vi "PickAndPlace_SiAndHB.vi"(0 "Operations":T1={"GoToTool"=TRUE, "PickTool"=TRUE, "GoToHB"=TRUE, "PickHB"=TRUE, "GoToSi"=TRUE, "PickSi"=TRUE, "GoToBP"=TRUE, "DropTool"=TRUE}, 1 "VacuumStates":path=path "C:/Users/TTUHEP/Documents/LabVIEW/GantryPrograms/Configs/PickPlaceVacuumStates.json", 5 "AssmbType":enum16{"BothSiHB", "Sensor", "HB"}(ring), 7 "Zone":enum16{"ZoneA", "ZoneB", "ZoneC", "ZoneD"}(ring), 9 "Position":enum16{"1", "2"}(ring), 11 "Error In":errorcluster) -> (4 "Log":string, 15 "Error Out":errorcluster)   [LabVIEW 2021]
panel:
  in  "Si Delay (milliseconds)":u32=30000
  in  "FastZHBPick":dbl=65.0
  out "HBXYZU":dbl[](array[numeric])
  out "Assembly_XYZU":dbl[](array[numeric])
  out "PUT_XYZU":dbl[](array[numeric])
  out "PUT rotation":dbl
  in  "FastZDrop":dbl=65.0
  in  "FastZToolPick":dbl=85.0
  in  "FastZSiPick":dbl=65.0
  in  "LineNo":u8
  in  "ZSpeed":dbl=10.0
  in  "XYSpeed":dbl=100.0
  out "SiXYZU":dbl[](array[numeric])
  out "ZoneBasedFileNameStarting":string
  in  "HB_PositionPartialFileName":string="HB_Position.txt"
  in  "SiPositionPartialFileName":string="Si_Position.txt"
  in  "PUT_PositionPartialFileName":string="PUT_Position.txt"
  in  "AssemblyPositionPartialFileName":string="BP_Position.txt"
  in  "BaseDirectory":string="C:\\Users\\TTUHEP\\Documents\\LabVIEW\\GantryPrograms\\Configs\\"
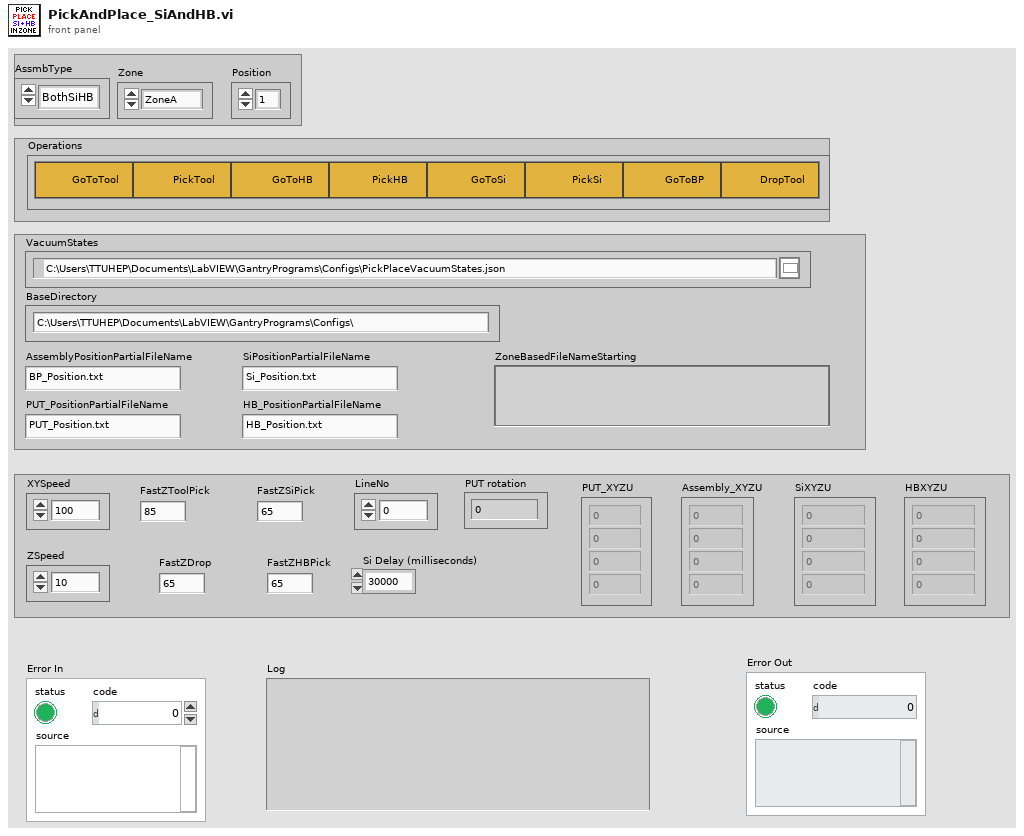
[diagram p1: front panel]
types:
  T1 = cluster{"GoToTool":bool, "PickTool":bool, "GoToHB":bool, "PickHB":bool, "GoToSi":bool, "PickSi":bool, "GoToBP":bool, "DropTool":bool}
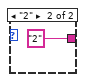
[diagram p2: hidden frame]
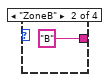
[diagram p3: hidden frame]
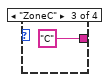
[diagram p4: hidden frame]
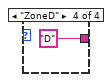
[diagram p5: hidden frame]
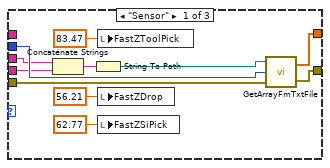
[diagram p6: hidden frame]
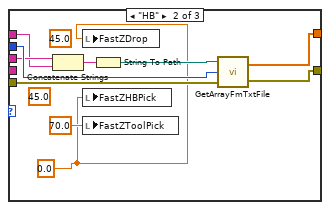
[diagram p7: hidden frame]
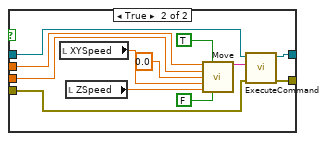
[diagram p8: hidden frame]
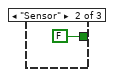
[diagram p10: hidden frame]
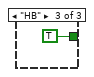
[diagram p11: hidden frame]
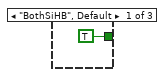
[diagram p14: hidden frame]
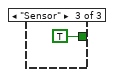
[diagram p15: hidden frame]
diagram:
  n1 = flat-sequence {
    tunnel: "Position" -> [w41]
    tunnel: "Zone" -> [w42]
    tunnel: [w42] -> w7
    tunnel: [w41] -> w6
    tunnel: [u8 0 ("LineNo")] -> w25
    tunnel: [w44] -> w17
    tunnel: ["Error In"] -> w16
    tunnel: w7 -> [w51]
    tunnel: w6 -> [w50]
    tunnel: [w64] -> w26
    tunnel: w25 -> [w63]
    tunnel: [w63] -> w23
    tunnel: w17 -> [w62]
    tunnel: w16 -> [w59]
    tunnel: [w118] -> w40
    tunnel: [w117] -> w39
    tunnel: [w116] -> w38
    tunnel: w26 -> [w114]
    tunnel: w23 -> [w115]
    tunnel: w40 -> [w145]
    tunnel: w39 -> [w144]
    tunnel: w38 -> [w143]
    tunnel: [w142] -> w37
    tunnel: [w141] -> w36
    tunnel: w37 -> [w151]
    tunnel: w36 -> [w150]
    tunnel: [w149] -> w35
    tunnel: [w148] -> w34
    tunnel: w35 -> [w189]
    tunnel: w34 -> [w188]
    tunnel: [w180] -> w5
    tunnel: [w179] -> w3
    tunnel: [w178] -> w2
    tunnel: [w215] -> w33
    tunnel: [w216] -> w32
    tunnel: w5 -> [w217]
    tunnel: [w217] -> w4
    tunnel: w3 -> [w216]
    tunnel: w2 -> [w215]
    tunnel: w33 -> [w225]
    tunnel: w32 -> [w224]
    tunnel: [w223] -> w11
    tunnel: [w222] -> w9
    tunnel: w4 -> [w220]
    tunnel: w11 -> [w262]
    tunnel: [w262] -> w10
    tunnel: w9 -> [w263]
    tunnel: [w263] -> w8
    tunnel: w10 -> [w272]
    tunnel: [w270] -> w15
    tunnel: w8 -> [w271]
    tunnel: [w269] -> w14
    tunnel: [w264] -> w1
    tunnel: w15 -> [w307]
    tunnel: w14 -> [w306]
    tunnel: [w303] -> w13
    tunnel: [w302] -> w12
    tunnel: w1 -> [w299]
    tunnel: w13 -> [w354]
    tunnel: [w352] -> w31
    tunnel: [w351] -> w30
    tunnel: [w350] -> w29
    tunnel: w12 -> [w355]
    tunnel: w31 -> [w382]
    tunnel: w30 -> [w381]
    tunnel: w29 -> [w379]
    tunnel: [w377] -> w28
    tunnel: [w376] -> w27
    tunnel: w28 -> [w388]
    tunnel: w27 -> [w387]
    tunnel: [w386] -> w21
    tunnel: [w385] -> w20
    tunnel: w21 -> [w426]
    tunnel: w20 -> [w425]
    tunnel: [w424] -> w18
    tunnel: [w431] -> w19
    tunnel: w18 -> [w429]
    frame #0 {
    }
    frame #1 {
      n2 = case shown="\"ZoneA\", Default" w51 {
        tunnel: ["A" "B" "C" "D"] -> w47
        frame "ZoneA", Default {
        }
        frame "ZoneB" {
        }
        frame "ZoneC" {
        }
        frame "ZoneD" {
        }
      }
      n3 = case shown="\"1\", Default" w50 {
        tunnel: ["1" "2"] -> w46
        frame "1", Default {
        }
        frame "2" {
        }
      }
      n4 = Concatenate Strings(w47, w46, "_" ("string")) -> (w49:string)
      n5 = Concatenate Strings("BaseDirectory", w49) -> (w44:string)
      "ZoneBasedFileNameStarting" <- w44
    }
    frame #2 {
      n6 = case shown="\"BothSiHB\", Default" "AssmbType" {
        tunnel: w63 -> [w77 w87 w92]
        tunnel: [w76 w86 w103] -> w66
        tunnel: w59 -> [w75 w85 w102]
        tunnel: [w74 w84 w90] -> w64
        tunnel: w62 -> [w70 w82 w94]
        tunnel: "SiPositionPartialFileName" -> [w67 _ w97]
        tunnel: "HB_PositionPartialFileName" -> [_ w79 w93]
        frame "Sensor" {
          n7 = Concatenate Strings(w70, w67) -> (w69:string)
          n8 = String To Path(string=w69) -> (path=w68:path)
          n9 = local write "FastZToolPick"(83.47 ("FastZToolPick")) -> ()
          n10 = local write "FastZDrop"(56.21 ("FastZDrop")) -> ()
          n11 = local write "FastZSiPick"(62.77 ("FastZSiPCBPick")) -> ()
          n12 = call "GetArrayFmTxtFile.vi"("error in"=w75, "LineNo."=w77, "TextFile"=w68) -> ("error out"=w74:errorcluster, "Array"=w76:dbl[])
        }
        frame "HB" {
          w78 = 0.0
          (unwired) 45.0 ("FastZDrop")
          (unwired) 45.0 ("FastZSiPCBPick")
          n13 = Concatenate Strings(w82, w79) -> (w81:string)
          n14 = local write "FastZDrop"(w78) -> ()
          n15 = local write "FastZHBPick"(w78) -> ()
          n16 = local write "FastZToolPick"(70.0 ("FastZToolPick")) -> ()
          n17 = String To Path(string=w81) -> (path=w80:path)
          n18 = call "GetArrayFmTxtFile.vi"("error in"=w85, "LineNo."=w87, "TextFile"=w80) -> ("error out"=w84:errorcluster, "Array"=w86:dbl[])
        }
        frame "BothSiHB", Default {
          w88 = 0.0
          (unwired) 45.0 ("FastZSiPCBPick")
          (unwired) 48.0 ("FastZDrop")
          n19 = Concatenate Strings(w94, w93) -> (w96:string)
          n20 = Concatenate Strings(w94, w97) -> (w99:string)
          n21 = local write "FastZSiPick"(60.0 ("FastZSiPCBPick")) -> ()
          n22 = local write "FastZToolPick"(80.0 ("FastZToolPick")) -> ()
          n23 = local write "FastZHBPick"(w88) -> ()
          n24 = local write "FastZDrop"(w88) -> ()
          n25 = String To Path(string=w96) -> (path=w95:path)
          n26 = String To Path(string=w99) -> (path=w98:path)
          n27 = call "GetArrayFmTxtFile.vi"("error in"=w102, "LineNo."=w92, "TextFile"=w98) -> ("error out"=w91:errorcluster, "Array"=w103:dbl[])
          n28 = call "GetArrayFmTxtFile.vi"("error in"=w91, "LineNo."=w92, "TextFile"=w95) -> ("error out"=w90:errorcluster, "Array"=→"HBXYZU":dbl[])
        }
      }
      "SiXYZU" <- w66
    }
    frame #3 {
      n29 = local read "ZoneBasedFileNameStarting"() -> (w110:string)
      n30 = Concatenate Strings(w110, "PUT_PositionPartialFileName") -> (w109:string)
      n31 = String To Path(string=w109) -> (path=w108:path)
      n32 = call "GetArrayFmTxtFile.vi"("error in"=w114, "LineNo."=w115, "TextFile"=w108) -> ("error out"=w107:errorcluster, "Array"=w112:dbl[])
      "PUT_XYZU" <- w112
      n33 = local read "Operations"() -> (w105:T1)
      n34 = call "Connect.vi"("error in (no error)"=w107) -> ("error out"=w106:errorcluster, "controller"=w113:refnum<k24>)  [unwired: 9 in]
      n35 = Index Array(array=w112, index=3) -> (element=w116:dbl)
      "PUT rotation" <- w116
      n36 = Index Array(array=w112, index=0) -> (element=w120:dbl)
      n37 = Index Array(array=w112, index=1) -> (element=w119:dbl)
      n38 = Unbundle By Name(w105) -> ("GoToTool"=w104:bool)
      n39 = call "ExecuteCommand.vi"("error in (no error)"=w106, "Command Code"="G90\nG1 Z0 F50", "controller in"=w113) -> ("error out"=w126:errorcluster, "controller out"=w125:refnum<k24>)  [unwired: 6 in, 1 out]
      n40 = case shown="False" w104 {
        tunnel: w125 -> [w128 w137]
        tunnel: w126 -> [w127 w136]
        tunnel: [w127 w135] -> w118
        tunnel: [w128 w134] -> w117
        tunnel: w120 -> [_ w133]
        tunnel: w119 -> [_ w132]
        frame False {
        }
        frame True {
          n41 = local read "XYSpeed"() -> (w130:dbl)
          n42 = local read "ZSpeed"() -> (w129:dbl)
          n43 = call "Move.vi"("X"=w133, "Absolute"=TRUE, "Y"=w132, "Z"=0.0, "SpeedXY (mm/s)"=w130, "SpeedZ (mm/s)"=w129, "Move Z first"=FALSE) -> ("Position Gcode"=w138:string)  [unwired: 8 in]
          n44 = call "ExecuteCommand.vi"("error in (no error)"=w136, "Command Code"=w138, "controller in"=w137) -> ("error out"=w135:errorcluster, "controller out"=w134:refnum<k24>)  [unwired: 6 in, 1 out]
        }
      }
    }
    frame #4 {
      n45 = call "RotateGH_U.vi"("error in (no error)"=w145, "controller in"=w144, "U"=w143) -> ("error out"=w142:errorcluster, "controller out"=w141:refnum<k24>)
    }
    frame #5 {
      n46 = local read "Operations"() -> (w146:T1)
      n47 = Unbundle By Name(w146) -> ("PickTool"=w147:bool)
      n48 = case shown="True" w147 {
        tunnel: w151 -> [w153 w162]
        tunnel: w150 -> [w152 w175]
        tunnel: [w153 w154] -> w149
        tunnel: [w152 w158] -> w148
        frame False {
        }
        frame True {
          w165 = u8 0
          n49 = call "JSONfileReader.vi"("error in"=w162, "Variant"=w165, "ItemName"="PickTool", "FileIn"="VacuumStates") -> ("error out"=w160:errorcluster, "Data"=w164:variant, "Found"=w169:bool)
          n50 = Not(x=w169) -> (.not. x?=w170:bool)
          n51 = Variant To Data(error in=w160, type=w165, Variant=w164) -> (data=w163:u8, error out=w159:errorcluster)
          n52 = local read "FastZToolPick"() -> (w157:dbl)
          n53 = local read "Position"() -> (w174:enum16{"1", "2"})
          n54 = call "AddError.vi"("NoErrorMessage"="Vac OK", "ErrorMessage"="Could not get vacuum state from json file.", "error in"=w159, "code"=-998, "Error?"=w170) -> ("Error out"=w161:errorcluster)  [unwired: 6 in]
          n55 = local read "Zone"() -> (w173:enum16{"ZoneA", "ZoneB", "ZoneC", "ZoneD"})
          n56 = call "ZoneVacCtrldPickDrop.vi"("Position"=w174, "Zone"=w173, "VacuumState"=w163, "error in (no error)"=w161, "controller in"=w175, "Zspeed"=50.0, "Z"=w157) -> ("error out"=w155:errorcluster, "controller out"=w158:refnum<k24>)  [unwired: 3 in]
          n57 = call <vilib>:"Simple Error Handler.vi"("error in (no error)"=w155) -> ("error?"=w156:bool, "error out"=w154:errorcluster)  [unwired: 4 in, 3 out]
          n58 = Stop(stop? (T)=w156) -> ()
        }
      }
    }
    frame #6 {
      n59 = local read "AssmbType"() -> (w183:enum16{"BothSiHB", "Sensor", "HB"})
      n60 = case shown="\"BothSiHB\", Default" w183 {
        tunnel: [TRUE FALSE TRUE] -> w180
        frame "BothSiHB", Default {
        }
        frame "Sensor" {
        }
        frame "HB" {
        }
      }
      n61 = local read "Operations"() -> (w184:T1)
      n62 = local read "HBXYZU"() -> (w187:dbl[])
      n63 = local read "PUT rotation"() -> (w186:dbl)
      n64 = Unbundle By Name(w184) -> ("GoToHB"=w182:bool)
      n65 = Index Array(array=w187, index=3) -> (element=w185:dbl)
      n66 = Index Array(array=w187, index=0) -> (element=w193:dbl)
      n67 = Index Array(array=w187, index=1) -> (element=w194:dbl)
      n68 = Add(x=w186, y=w185) -> (x+y=w177:dbl)
      n69 = And(x=w182, y=w180) -> (x .and. y?=w181:bool)
      n70 = case shown="True" w181 {
        tunnel: w188 -> [w199 w211]
        tunnel: w189 -> [w198 w210]
        tunnel: w193 -> [_ w209]
        tunnel: w194 -> [_ w208]
        tunnel: [w198 w204] -> w179
        tunnel: [w199 w203] -> w178
        tunnel: w177 -> [_ w202]
        frame False {
        }
        frame True {
          n71 = local read "XYSpeed"() -> (w205:dbl)
          n72 = local read "ZSpeed"() -> (w206:dbl)
          n73 = call "Move.vi"("X"=w209, "Absolute"=TRUE, "Y"=w208, "Z"=0.0, "SpeedXY (mm/s)"=w205, "SpeedZ (mm/s)"=w206, "Move Z first"=FALSE) -> ("Position Gcode"=w212:string)  [unwired: 8 in]
          n74 = call "ExecuteCommand.vi"("error in (no error)"=w210, "Command Code"=w212, "controller in"=w211) -> ("error out"=w200:errorcluster, "controller out"=w201:refnum<k24>)  [unwired: 6 in, 1 out]
          n75 = call "RotateGH_U.vi"("error in (no error)"=w200, "controller in"=w201, "U"=w202) -> ("error out"=w204:errorcluster, "controller out"=w203:refnum<k24>)
        }
      }
    }
    frame #7 {
    }
    frame #8 {
      n76 = local read "Operations"() -> (w221:T1)
      n77 = Unbundle By Name(w221) -> ("PickHB"=w218:bool)
      n78 = And(x=w220, y=w218) -> (x .and. y?=w219:bool)
      n79 = case shown="True" w219 {
        tunnel: w224 -> [w227 w248]
        tunnel: w225 -> [w226 w242]
        tunnel: [w227 w245] -> w222
        tunnel: [w226 w244] -> w223
        frame False {
        }
        frame True {
          w236 = u8 0
          w251 = u8 0
          w229 = "Could not get vacuum state from json file." ("ErrorMessage")
          n80 = local read "VacuumStates"() -> (w232:path)
          n81 = call "JSONfileReader.vi"("error in"=w248, "Variant"=w251, "ItemName"="PickHB", "FileIn"=w232) -> ("error out"=w247:errorcluster, "Data"=w250:variant, "Found"=w254:bool)
          n82 = Not(x=w254) -> (.not. x?=w255:bool)
          n83 = Variant To Data(error in=w247, type=w251, Variant=w250) -> (data=w249:u8, error out=w246:errorcluster)
          n84 = call "AddError.vi"("NoErrorMessage"="Vac OK", "ErrorMessage"=w229, "error in"=w246, "code"=-998, "Error?"=w255) -> ("Error out"=w231:errorcluster)  [unwired: 6 in]
          n85 = call "JSONfileReader.vi"("error in"=w231, "Variant"=w236, "ItemName"="ReleaseHB", "FileIn"=w232) -> ("error out"=w234:errorcluster, "Data"=w235:variant, "Found"=w239:bool)
          n86 = Not(x=w239) -> (.not. x?=w240:bool)
          n87 = Variant To Data(error in=w234, type=w236, Variant=w235) -> (data=w228:u8, error out=w233:errorcluster)
          n88 = local read "FastZHBPick"() -> (w243:dbl)
          n89 = local read "Position"() -> (w258:enum16{"1", "2"})
          n90 = call "AddError.vi"("NoErrorMessage"="Vac OK", "ErrorMessage"=w229, "error in"=w233, "code"=-998, "Error?"=w240) -> ("Error out"=w230:errorcluster)  [unwired: 6 in]
          n91 = local read "Zone"() -> (w257:enum16{"ZoneA", "ZoneB", "ZoneC", "ZoneD"})
          n92 = call "ZoneVacCtrldPickDrop_2StepVac.vi"("Position"=w258, "VacuumState2"=w228, "Zone"=w257, "VacuumState1"=w249, "error in (no error)"=w230, "controller in"=w242, "Zspeed"=50.0, "Z"=w243) -> ("error out"=w245:errorcluster, "controller out"=w244:refnum<k24>)  [unwired: 2 in]
        }
      }
    }
    frame #9 {
      n93 = One Button Dialog(message="Removed tape on HB?", button name ("OK")="Yes" ("T button name (\"OK\")")) -> ()  [unwired: 1 out]
    }
    frame #10 {
      n94 = local read "AssmbType"() -> (w267:enum16{"BothSiHB", "Sensor", "HB"})
      n95 = local read "Operations"() -> (w268:T1)
      n96 = case shown="\"HB\"" w267 {
        tunnel: [TRUE FALSE TRUE] -> w265
        frame "BothSiHB", Default {
        }
        frame "HB" {
        }
        frame "Sensor" {
        }
      }
      n97 = Unbundle By Name(w268) -> ("GoToSi"=w266:bool)
      n98 = And(x=w266, y=w265) -> (x .and. y?=w264:bool)
      n99 = case shown="True" w264 {
        tunnel: w272 -> [w277 w289]
        tunnel: w271 -> [w276 w288]
        tunnel: [w277 w284] -> w270
        tunnel: [w276 w283] -> w269
        frame False {
        }
        frame True {
          n100 = local read "SiXYZU"() -> (w279:dbl[])
          n101 = local read "PUT rotation"() -> (w278:dbl)
          n102 = local read "XYSpeed"() -> (w281:dbl)
          n103 = local read "ZSpeed"() -> (w280:dbl)
          n104 = Index Array(array=w279, index=3) -> (element=w287:dbl)
          n105 = Index Array(array=w279, index=0) -> (element=w292:dbl)
          n106 = Index Array(array=w279, index=1) -> (element=w291:dbl)
          n107 = Add(x=w278, y=w287) -> (x+y=w286:dbl)
          n108 = call "Move.vi"("X"=w292, "Absolute"=TRUE, "Y"=w291, "Z"=0.0, "SpeedXY (mm/s)"=w281, "SpeedZ (mm/s)"=w280, "Move Z first"=FALSE) -> ("Position Gcode"=w296:string)  [unwired: 8 in]
          n109 = call "ExecuteCommand.vi"("error in (no error)"=w288, "Command Code"=w296, "controller in"=w289) -> ("error out"=w282:errorcluster, "controller out"=w285:refnum<k24>)  [unwired: 6 in, 1 out]
          n110 = call "RotateGH_U.vi"("error in (no error)"=w282, "controller in"=w285, "U"=w286) -> ("error out"=w283:errorcluster, "controller out"=w284:refnum<k24>)
        }
      }
    }
    frame #11 {
      n111 = local read "Operations"() -> (w304:T1)
      n112 = local read "VacuumStates"() -> (w305:path)
      n113 = Unbundle By Name(w304) -> ("PickSi"=w300:bool)
      n114 = And(x=w300, y=w299) -> (x .and. y?=w301:bool)
      n115 = case shown="True" w301 {
        tunnel: w306 -> [w309 w333]
        tunnel: w307 -> [w308 w328]
        tunnel: [w309 w330] -> w303
        tunnel: [w308 w329] -> w302
        tunnel: w305 -> [_ w314]
        frame False {
        }
        frame True {
          w322 = u8 0
          w336 = u8 0
          w316 = "Could not get vacuum state from json file." ("ErrorMessage")
          n116 = call "JSONfileReader.vi"("error in"=w333, "Variant"=w336, "ItemName"="PickSi", "FileIn"=w314) -> ("error out"=w332:errorcluster, "Data"=w335:variant, "Found"=w339:bool)
          n117 = Not(x=w339) -> (.not. x?=w340:bool)
          n118 = Variant To Data(error in=w332, type=w336, Variant=w335) -> (data=w334:u8, error out=w331:errorcluster)
          n119 = call "AddError.vi"("NoErrorMessage"="Vac OK", "ErrorMessage"=w316, "error in"=w331, "code"=-998, "Error?"=w340) -> ("Error out"=w318:errorcluster)  [unwired: 6 in]
          n120 = call "JSONfileReader.vi"("error in"=w318, "Variant"=w322, "ItemName"="ReleaseSi", "FileIn"=w314) -> ("error out"=w320:errorcluster, "Data"=w321:variant, "Found"=w325:bool)
          n121 = Not(x=w325) -> (.not. x?=w326:bool)
          n122 = Variant To Data(error in=w320, type=w322, Variant=w321) -> (data=w315:u8, error out=w319:errorcluster)
          n123 = local read "FastZSiPick"() -> (w311:dbl)
          n124 = local read "Position"() -> (w312:enum16{"1", "2"})
          n125 = call "AddError.vi"("NoErrorMessage"="Vac OK", "ErrorMessage"=w316, "error in"=w319, "code"=-998, "Error?"=w326) -> ("Error out"=w317:errorcluster)  [unwired: 6 in]
          n126 = local read "Zone"() -> (w313:enum16{"ZoneA", "ZoneB", "ZoneC", "ZoneD"})
          n127 = call "ZoneVacCtrldPickDrop_2StepVac.vi"("milliseconds to wait"="Si Delay (milliseconds)", "Position"=w312, "VacuumState2"=w315, "Zone"=w313, "VacuumState1"=w334, "error in (no error)"=w317, "controller in"=w328, "Zspeed"=50.0, "Z"=w311) -> ("error out"=w330:errorcluster, "controller out"=w329:refnum<k24>)  [unwired: 1 in]
        }
      }
    }
    frame #12 {
      n128 = local read "ZoneBasedFileNameStarting"() -> (w348:string)
      n129 = Concatenate Strings(w348, "AssemblyPositionPartialFileName") -> (w346:string)
      n130 = local read "LineNo"() -> (w356:u8)
      n131 = String To Path(string=w346) -> (path=w345:path)
      n132 = local read "Operations"() -> (w344:T1)
      n133 = call "GetArrayFmTxtFile.vi"("error in"=w354, "LineNo."=w356, "TextFile"=w345) -> ("error out"=w353:errorcluster, "Array"=w349:dbl[])
      "Assembly_XYZU" <- w349
      n134 = Unbundle By Name(w344) -> ("GoToBP"=w343:bool)
      n135 = Index Array(array=w349, index=3) -> (element=w350:dbl)
      n136 = Index Array(array=w349, index=0) -> (element=w361:dbl)
      n137 = Index Array(array=w349, index=1) -> (element=w360:dbl)
      n138 = case shown="True" w343 {
        tunnel: w355 -> [w363 w372]
        tunnel: w353 -> [w362 w371]
        tunnel: [w362 w370] -> w352
        tunnel: [w363 w369] -> w351
        tunnel: w361 -> [_ w368]
        tunnel: w360 -> [_ w367]
        frame False {
        }
        frame True {
          n139 = local read "XYSpeed"() -> (w364:dbl)
          n140 = local read "ZSpeed"() -> (w365:dbl)
          n141 = call "Move.vi"("X"=w368, "Absolute"=TRUE, "Y"=w367, "Z"=0.0, "SpeedXY (mm/s)"=w364, "SpeedZ (mm/s)"=w365, "Move Z first"=FALSE) -> ("Position Gcode"=w373:string)  [unwired: 8 in]
          n142 = call "ExecuteCommand.vi"("error in (no error)"=w371, "Command Code"=w373, "controller in"=w372) -> ("error out"=w370:errorcluster, "controller out"=w369:refnum<k24>)  [unwired: 6 in, 1 out]
        }
      }
    }
    frame #13 {
      n143 = local read "PUT rotation"() -> (w380:dbl)
      n144 = Add(x=w380, y=w379) -> (x+y=w378:dbl)
      n145 = call "RotateGH_U.vi"("error in (no error)"=w382, "controller in"=w381, "U"=w378) -> ("error out"=w377:errorcluster, "controller out"=w376:refnum<k24>)
    }
    frame #14 {
      n146 = local read "Operations"() -> (w384:T1)
      n147 = Unbundle By Name(w384) -> ("DropTool"=w383:bool)
      n148 = case shown="True" w383 {
        tunnel: w388 -> [w390 w408]
        tunnel: w387 -> [w389 w407]
        tunnel: [w390 w406] -> w386
        tunnel: [w389 w405] -> w385
        frame False {
        }
        frame True {
          w399 = u8 0
          w414 = u8 0
          n149 = local read "VacuumStates"() -> (w394:path)
          n150 = call "JSONfileReader.vi"("error in"=w408, "Variant"=w414, "ItemName"="HoldPUT", "FileIn"=w394) -> ("error out"=w421:errorcluster, "Data"=w419:variant, "Found"=w418:bool)
          n151 = Not(x=w418) -> (.not. x?=w417:bool)
          n152 = Variant To Data(error in=w421, type=w414, Variant=w419) -> (data=w420:u8, error out=w422:errorcluster)
          n153 = call "AddError.vi"("NoErrorMessage"="Vac OK", "ErrorMessage"="Could not get vacuum state from json file.", "error in"=w422, "code"=-998, "Error?"=w417) -> ("Error out"=w393:errorcluster)  [unwired: 6 in]
          n154 = call "JSONfileReader.vi"("error in"=w393, "Variant"=w399, "ItemName"="DropTool", "FileIn"=w394) -> ("error out"=w403:errorcluster, "Data"=w402:variant, "Found"=w401:bool)
          n155 = Not(x=w401) -> (.not. x?=w400:bool)
          n156 = Variant To Data(error in=w403, type=w399, Variant=w402) -> (data=w391:u8, error out=w404:errorcluster)
          n157 = local read "FastZDrop"() -> (w423:dbl)
          n158 = local read "Position"() -> (w415:enum16{"1", "2"})
          n159 = call "AddError.vi"("NoErrorMessage"="Vac OK", "ErrorMessage"="Could not get vacuum state from json file.", "error in"=w404, "code"=-998, "Error?"=w400) -> ("Error out"=w392:errorcluster)  [unwired: 6 in]
          n160 = local read "Zone"() -> (w416:enum16{"ZoneA", "ZoneB", "ZoneC", "ZoneD"})
          n161 = call "ZoneVacCtrldPickDrop_2StepVac.vi"("Position"=w415, "VacuumState2"=w391, "Zone"=w416, "VacuumState1"=w420, "error in (no error)"=w392, "controller in"=w407, "Zspeed"=50.0, "Z"=w423) -> ("error out"=w406:errorcluster, "controller out"=w405:refnum<k24>)  [unwired: 2 in]
        }
      }
    }
    frame #15 {
      n162 = call "Disconnect.vi"("error in (no error)"=w426, "controller"=w425) -> ("error out"=w424:errorcluster)  [unwired: 9 in]
    }
    frame #16 {
      n163 = flat-sequence {
        tunnel: [w437] -> w430
        tunnel: w429 -> [w437]
        tunnel: [w440] -> w436
        tunnel: w430 -> [w439]
        tunnel: w436 -> [w448]
        tunnel: [w447] -> w435
        tunnel: [w456] -> w434
        tunnel: w435 -> [w457]
        tunnel: w434 -> [w464]
        tunnel: [w463] -> w433
        tunnel: [w471] -> w432
        tunnel: w433 -> [w471]
        tunnel: [w479] -> w428
        tunnel: w432 -> [w479]
        tunnel: w428 -> [w494]
        tunnel: [w494] -> w427
        tunnel: [w495] -> w431
        tunnel: w427 -> [w495]
        frame #0 {
          "Log" <- ""
        }
        frame #1 {
          n164 = local read "AssmbType"() -> (w446:enum16{"BothSiHB", "Sensor", "HB"})
          n165 = local read "Log"() -> (w441:string)
          n166 = Format Into String(initial string="AssemblyType: ", error in=w439, w446) -> (resulting string=w443:string, error out=w440:errorcluster)  [unwired: 1 in]
          n167 = Concatenate Strings(w441, w443, "\r\n") -> (w445:string)
          n168 = local write "Log"(w445) -> ()
        }
        frame #2 {
          n169 = local read "Zone"() -> (w454:enum16{"ZoneA", "ZoneB", "ZoneC", "ZoneD"})
          n170 = local read "Log"() -> (w451:string)
          n171 = Format Into String(initial string="Zone: ", error in=w448, w454) -> (resulting string=w453:string, error out=w447:errorcluster)  [unwired: 1 in]
          n172 = Concatenate Strings(w451, w453, "\r\n") -> (w452:string)
          n173 = local write "Log"(w452) -> ()
        }
        frame #3 {
          n174 = local read "Position"() -> (w460:enum16{"1", "2"})
          n175 = local read "Log"() -> (w462:string)
          n176 = Format Into String(initial string="AssemblyPosition: ", error in=w457, w460) -> (resulting string=w461:string, error out=w456:errorcluster)  [unwired: 1 in]
          n177 = Concatenate Strings(w462, w461, "\r\n") -> (w455:string)
          n178 = local write "Log"(w455) -> ()
        }
        frame #4 {
          n179 = local read "LineNo"() -> (w470:u8)
          n180 = local read "Log"() -> (w468:string)
          n181 = Format Into String(initial string="ComponentPosTexFileLineNo: ", error in=w464, w470) -> (resulting string=w469:string, error out=w463:errorcluster)  [unwired: 1 in]
          n182 = Concatenate Strings(w468, w469, "\r\n") -> (w467:string)
          n183 = local write "Log"(w467) -> ()
        }
        frame #5 {
          n184 = local read "PUT_XYZU"() -> (w478:dbl[])
          n185 = Array To Spreadsheet String(delimiter (Tab)=",", array=w478, 3:"%f" ("format string")) -> (spreadsheet string=w475:string)
          n186 = local read "Log"() -> (w473:string)
          n187 = Concatenate Strings(w473, "PUT_XYZU: " ("string"), w475) -> (w474:string)
          n188 = local write "Log"(w474) -> ()
        }
        frame #6 {
          n189 = local read "HBXYZU"() -> (w486:dbl[])
          n190 = Array To Spreadsheet String(delimiter (Tab)=",", array=w486, 3:"%f" ("format string")) -> (spreadsheet string=w483:string)
          n191 = local read "Log"() -> (w481:string)
          n192 = Concatenate Strings(w481, "HB_XYZU: " ("string"), w483) -> (w482:string)
          n193 = local write "Log"(w482) -> ()
        }
        frame #7 {
          n194 = local read "SiXYZU"() -> (w489:dbl[])
          n195 = Array To Spreadsheet String(delimiter (Tab)=",", array=w489, 3:"%f" ("format string")) -> (spreadsheet string=w491:string)
          n196 = local read "Log"() -> (w488:string)
          n197 = Concatenate Strings(w488, "Si_XYZU: " ("string"), w491) -> (w487:string)
          n198 = local write "Log"(w487) -> ()
        }
        frame #8 {
          n199 = local read "Assembly_XYZU"() -> (w496:dbl[])
          n200 = Array To Spreadsheet String(delimiter (Tab)=",", array=w496, 3:"%f" ("format string")) -> (spreadsheet string=w501:string)
          n201 = local read "Log"() -> (w497:string)
          n202 = Concatenate Strings(w497, "Assembly_XYZU: " ("string"), w501) -> (w499:string)
          n203 = local write "Log"(w499) -> ()
        }
      }
    }
  }
  "Error Out" <- w19
